vi "8.6CompatibleGlobalVar.vi"() -> ()   [LabVIEW 2012]
panel:
  out "8.6 compatible ?":bool
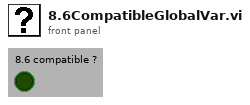
[diagram p1: front panel]
diagram:
